vi "Add Member Data to Private Data Control.vi"(7 "AppInst":refnum<vi>, 8 "error in (no error)":errorcluster, 9 "Controls":refnum<vi>[](array[refnum]), 10 "Target Path":path) -> (0 "error out":errorcluster)   [LabVIEW 2020, in "Message Maker.lvlib"]
uses:
  Message Maker.lvlib
  <vilib>/Utility/miscctls.llb/LVPositionTypeDef.ctl
  <vilib>/Utility/traverseref.llb/TRef TravTarget.ctl
  <vilib>/Utility/traverseref.llb/VI Scripting - Traverse.lvlib
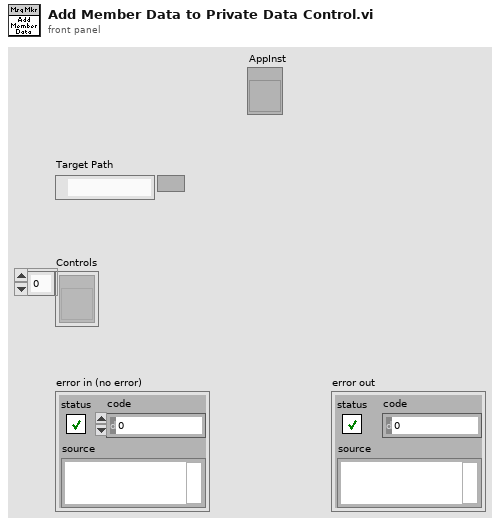
[diagram p1: front panel]
types:
  T1 = typedef "TRef TravTarget.ctl" = enum16{"FP", "BD", "Other"}
  T2 = enum32{"Invalid", "Standard", "Closed", "Hidden", "Minimized", "Maximized"}
  T3 = typedef "LVPositionTypeDef.ctl" = cluster{"Left":i32, "Top":i32}
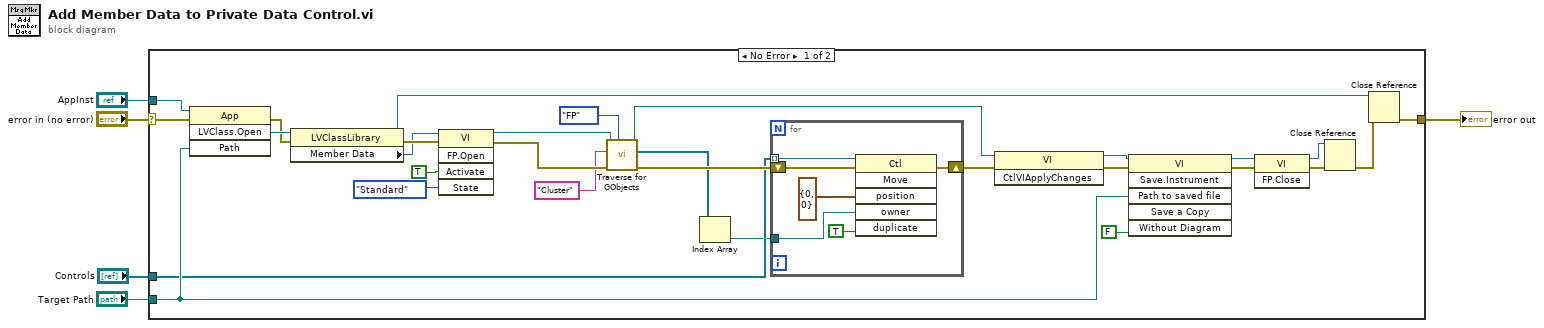
[diagram p0: block diagram]
diagram:
  n1 = case shown="No Error" "error in (no error)" {
    selector: "error in (no error)" -> [w21 w41]
    tunnel: [w30 w41] -> w5
    tunnel: "Target Path" -> [w22 _]
    tunnel: "AppInst" -> [w20 _]
    tunnel: "Controls" -> [w13 _]
    frame No Error {
      n2 = invoke class="App" method="LVClass.Open"(reference=w20, error in=w21, "Path"=w22) -> (error out=w32:errorcluster, "LVClass.Open"=w33:refnum<vi>)  [unwired: 1 in, 2 out]
      n3 = property class="LVClassLibrary"(reference=w33, error in=w32) -> (reference out=w17:refnum<vi>, error out=w16:errorcluster, "Member Data"=w15:refnum<vi>)
      n4 = invoke class="VI" method="FP.Open"(reference=w15, error in=w16, "Activate"=TRUE ("Activate?"), "State"=T2."Standard") -> (reference out=w10:refnum<vi>, error out=w25:errorcluster)  [unwired: 1 in, 3 out]
      n5 = call <vilib>:"Traverse for GObjects.vi"("Traverse Target"=TRef_TravTarget."FP", "error in (no error)"=w25, "Class Name"="Cluster", "VI Refnum"=w10) -> ("error out"=w14:errorcluster, "References"=w7:refnum<vi>[], "dup VI Refnum"=w6:refnum<vi>)  [unwired: 4 in, 1 out]
      n6 = Index Array(array=w7) -> (element=w11:refnum<vi>)  [unwired: 1 in]
      n7 = for {
        tunnel: w13 -> [w40] mode=indexing
        shift-right: [w37] -> w12
        shift-left: w14 -> [w38]
        tunnel: w11 -> [w35]
        n8 = invoke class="Ctl" method="Move"(reference=w40, error in=w38, "position"=T3 {"Left"=0, "Top"=0}, "owner"=w35, "duplicate"=TRUE ("Duplicate? (F)")) -> (error out=w37:errorcluster)  [unwired: 1 in, 5 out]
      }
      n9 = invoke class="VI" method="CtlVIApplyChanges"(reference=w6, error in=w12) -> (reference out=w18:refnum<vi>, error out=w19:errorcluster)  [unwired: 1 in, 1 out]
      n10 = invoke class="VI" method="Save.Instrument"(reference=w18, error in=w19, "Path to saved file"=w22, "Save a Copy"=FALSE) -> (reference out=w29:refnum<vi>, error out=w28:errorcluster)  [unwired: 2 in, 4 out]
      n11 = invoke class="VI" method="FP.Close"(reference=w29, error in=w28) -> (reference out=w26:refnum<vi>, error out=w27:errorcluster)  [unwired: 1 in, 1 out]
      n12 = Close Reference(reference=w26, error in (no error)=w27) -> (error out=w31:errorcluster)
      n13 = Close Reference(reference=w17, error in (no error)=w31) -> (error out=w30:errorcluster)
    }
    frame Error {
    }
  }
  "error out" <- w5
